vi "Climb_Set.vi"() -> ()   [LabVIEW 2018]
uses:
  <vilib>/Rock Robotics/WPI/DriverStation/WPI_DriverStationRobotMode2.ctl
  Climb_Control_Type.ctl
  Global_Variables/Climb_Globals.vi
  Global_Variables/Robot_Global_Data.vi
  Global_Variables/Sensor_Values.vi
  Global_Variables/Elevator_Globals.vi
  Global_Variables/Autonomous_Globals.vi
panel:
  in  "Climb_Position_Level_Two":dbl=13500.0
  in  "Climb_Level_Three_Position":dbl=34000.0
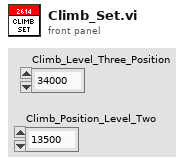
[diagram p1: front panel]
types:
  T1 = typedef "Climb_Control_Type.ctl" = enum16{"No_Op", "Brake", "Manual_Climb_Up", "Manual_Climb_Down", "Manual_Drive_Forward", "Manual_Drive_Backward", "Back_Wheels_Forward", "Lift_Retract", "Lift_Extend", "Extend_to_Second_Level", "Drop_Down", "Spin"}
  T2 = typedef "WPI_DriverStationRobotMode2.ctl" = enum16{"Autonomous Disabled", "Autonomous Enabled", "Teleop Disabled", "Teleop Enabled", "Disconnected", "Finish", "Test Disabled", "Test Enabled", "Emergency Stopped"}
  T3 = typedef "Climb_Notifier.ctl" = cluster{"Climb_Control_Type":T1, "Brake":bool, "Manual_Climb_Up":bool, "Manual_Drive_Forward":bool, "Manual_Drive_Backward":bool, "Manual_Climb_Down":bool, "Climb_Advance":bool, "Climb_Reverse":bool, "Parameter_One":dbl, "Parameter_Two":dbl, "Parameter_Three":dbl, "Step":i32, "Climb_Notifier":refnum<notifier>, "Climb_Distance":dbl, "Level_Two":bool, "Brake_State":bool, "Toggle_Servo":bool, "Drop_Back":bool}
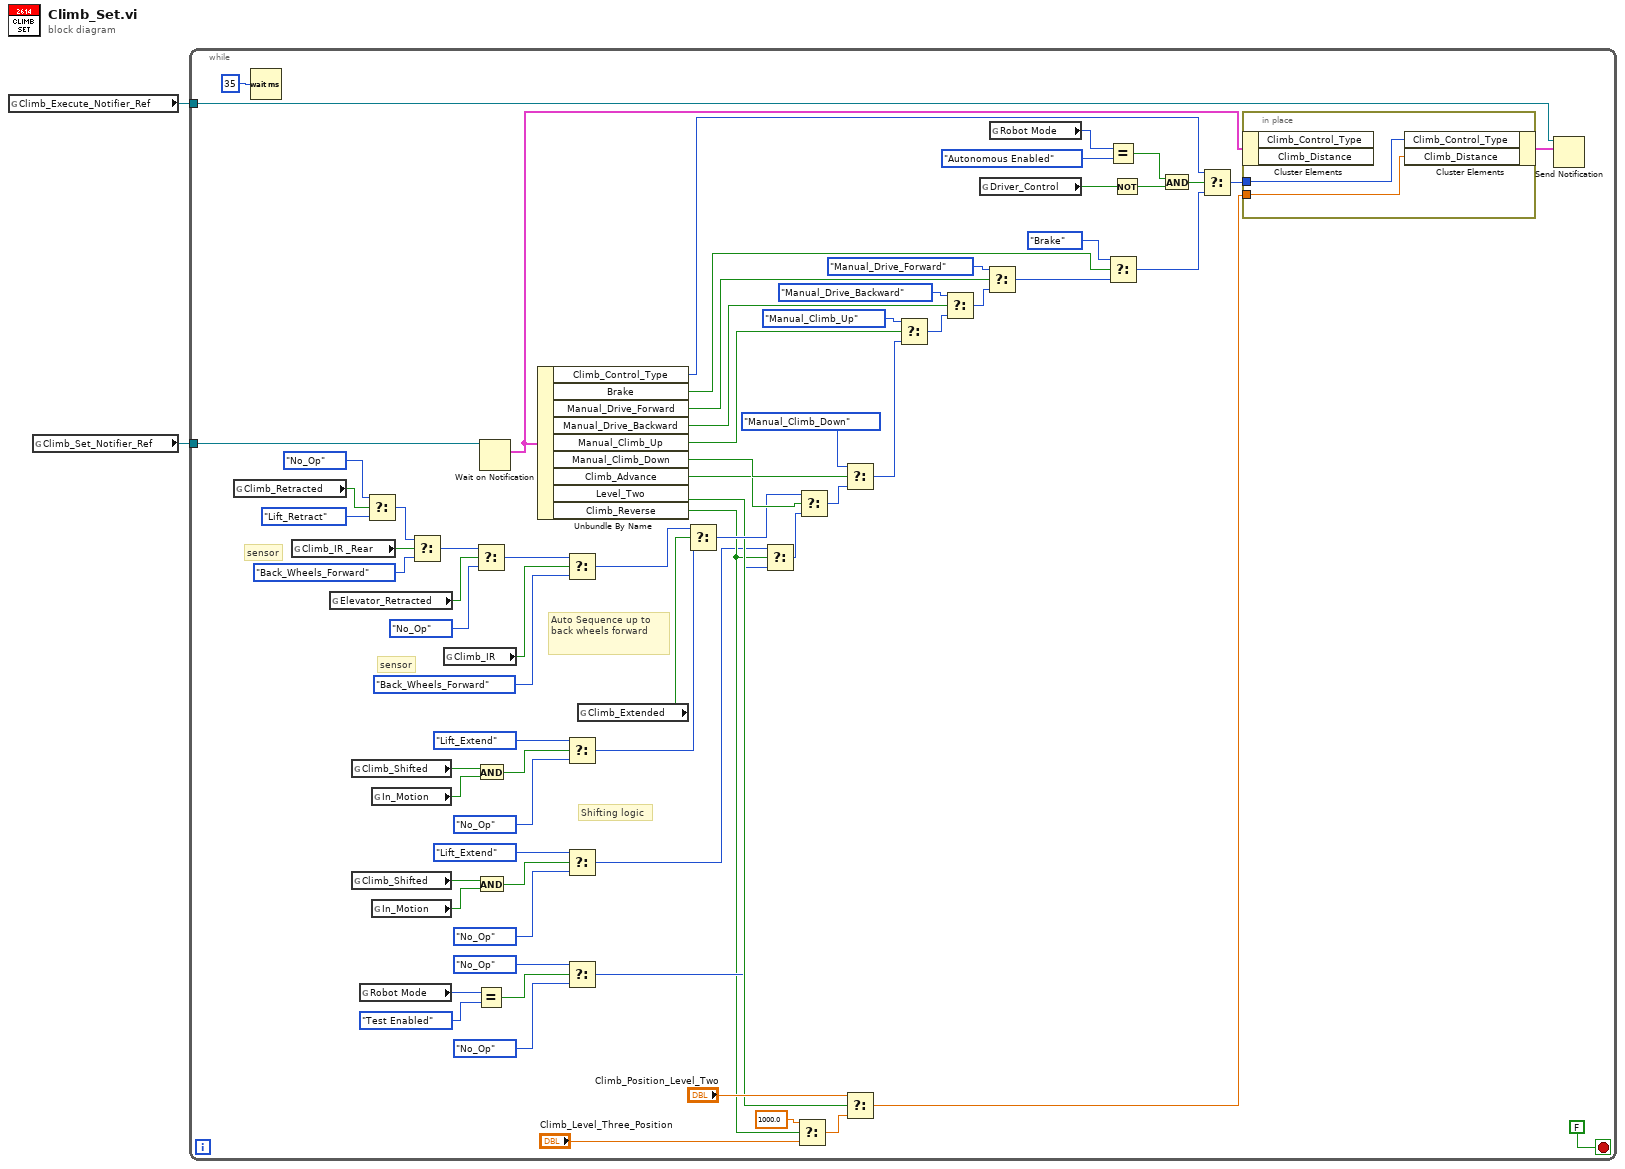
[diagram p0: block diagram]
diagram:
  n1 = global read "Climb_Globals.vi" "Climb_Execute_Notifier_Ref"() -> (w2:refnum<notifier>)
  n2 = global read "Climb_Globals.vi" "Climb_Set_Notifier_Ref"() -> (w1:refnum<notifier>)
  n3 = while {
    tunnel: w1 -> [w72]
    tunnel: w2 -> [w63]
    stop <- FALSE stop-if-true
    # "sensor"
    # "sensor"
    # "Shifting logic"
    # "Auto Sequence up to back wheels forward"
    n4 = global read "Climb_Globals.vi" "Climb_Retracted"() -> (w31:bool)
    n5 = Wait (ms)(milliseconds to wait=u32 35) -> ()  [unwired: 1 out]
    n6 = global read "Sensor_Values.vi" "Climb_IR _Rear"() -> (w33:bool)
    n7 = global read "Elevator_Globals.vi" "Elevator_Retracted"() -> (w37:bool)
    n8 = global read "Elevator_Globals.vi" "Climb_Shifted"() -> (w16:bool)
    n9 = global read "Elevator_Globals.vi" "Climb_Shifted"() -> (w7:bool)
    n10 = global read "Robot_Global_Data.vi" "Robot Mode"() -> (w65:T2)
    n11 = Select(t=Climb_Control_Type."No_Op", s=w31, f=Climb_Control_Type."Lift_Retract" ("t")) -> (s? t:f=w32:T1)
    n12 = global read "Sensor_Values.vi" "In_Motion"() -> (w15:bool)
    n13 = global read "Sensor_Values.vi" "In_Motion"() -> (w6:bool)
    n14 = Select(t=w32, s=w33, f=Climb_Control_Type."Back_Wheels_Forward" ("t")) -> (s? t:f=w35:T1)
    n15 = global read "Sensor_Values.vi" "Climb_IR"() -> (w39:bool)
    n16 = Select(t=w35, s=w37, f=Climb_Control_Type."No_Op") -> (s? t:f=w38:T1)
    n17 = Equal?(x=w65, y=WPI_DriverStationRobotMode2."Test Enabled") -> (x = y?=w64:bool)
    n18 = And(x=w16, y=w15) -> (x .and. y?=w14:bool)
    n19 = And(x=w7, y=w6) -> (x .and. y?=w5:bool)
    n20 = Wait on Notification(notifier=w72) -> (notification=w71:T3)  [unwired: 3 in, 3 out]
    n21 = Unbundle By Name(w71) -> ("Climb_Control_Type"=w67:T1, "Brake"=w62:bool, "Manual_Drive_Forward"=w55:bool, "Manual_Drive_Backward"=w58:bool, "Manual_Climb_Up"=w49:bool, "Manual_Climb_Down"=w48:bool, "Climb_Advance"=w44:bool, "Level_Two"=w26:bool, "Climb_Reverse"=w20:bool)
    n22 = Select(t=w38, s=w39, f=Climb_Control_Type."Back_Wheels_Forward") -> (s? t:f=w40:T1)
    n23 = Select(t=Climb_Control_Type."Lift_Extend", s=w14, f=Climb_Control_Type."No_Op") -> (s? t:f=w18:T1)
    n24 = Select(t=Climb_Control_Type."Lift_Extend", s=w5, f=Climb_Control_Type."No_Op") -> (s? t:f=w4:T1)
    n25 = Select(t=Climb_Control_Type."No_Op" ("Climb_Control_Type"), s=w64, f=Climb_Control_Type."No_Op" ("Climb_Control_Type")) -> (s? t:f=w25:T1)
    n26 = global read "Climb_Globals.vi" "Climb_Extended"() -> (w41:bool)
    n27 = Select(t=w40, s=w41, f=w18) -> (s? t:f=w43:T1)
    n28 = Select(t=w4, s=w20, f=w25) -> (s? t:f=w24:T1)
    n29 = Select(t=1000.0, s=w20, f="Climb_Level_Three_Position") -> (s? t:f=w23:dbl)
    n30 = Select(t=w43, s=w44, f=w24) -> (s? t:f=w45:T1)
    n31 = Select(t=Climb_Control_Type."Manual_Climb_Down", s=w48, f=w45) -> (s? t:f=w50:T1)
    n32 = Select(t="Climb_Position_Level_Two", s=w26, f=w23) -> (s? t:f=w28:dbl)
    n33 = Select(t=Climb_Control_Type."Manual_Climb_Up", s=w49, f=w50) -> (s? t:f=w51:T1)
    n34 = Select(t=Climb_Control_Type."Manual_Drive_Backward", s=w58, f=w51) -> (s? t:f=w57:T1)
    n35 = global read "Autonomous_Globals.vi" "Driver_Control"() -> (w11:bool)
    n36 = Select(t=Climb_Control_Type."Manual_Drive_Forward", s=w55, f=w57) -> (s? t:f=w56:T1)
    n37 = global read "Robot_Global_Data.vi" "Robot Mode"() -> (w69:T2)
    n38 = Equal?(x=w69, y=WPI_DriverStationRobotMode2."Autonomous Enabled") -> (x = y?=w10:bool)
    n39 = Select(t=Climb_Control_Type."Brake" ("Climb_Control_Type"), s=w62, f=w56) -> (s? t:f=w3:T1)
    n40 = Not(x=w11) -> (.not. x?=w12:bool)
    n41 = And(x=w10, y=w12) -> (x .and. y?=w13:bool)
    n42 = Select(t=w67, s=w13, f=w3) -> (s? t:f=w52:T1)
    n43 = in-place {
      in-place-border: w52 -> [w76]
      in-place-border: w28 -> [w75]
      n44 = in-place-cluster #1(w71) -> ()  [unwired: 2 out]
      n45 = in-place-cluster #1("Climb_Control_Type"=w76, "Climb_Distance"=w75) -> (w70:T3)
    }
    n46 = Send Notification(notification=w70, notifier=w63) -> ()  [unwired: 1 in, 2 out]
  }
